vi "Get Functions Name.vi"(8 "error in (no error)":errorcluster, 11 "QDDialogList in":refnum<class "QDDialogList.lvclass">) -> (0 "error out":errorcluster, 2 "Functions Name":string[](array[string]), 3 "QDDialogList out":refnum<class "QDDialogList.lvclass">)   [LabVIEW 2015, in "QDDialogList.lvclass"]
uses:
  QDDialogList.lvclass
  QDDialogList.lvclass/QDDialogList.ctl
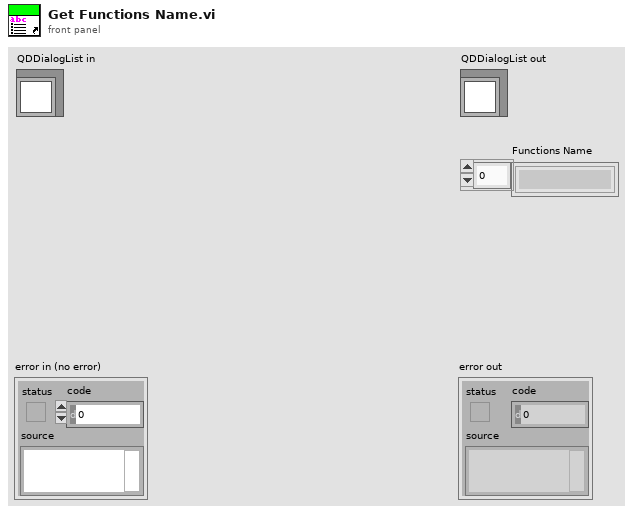
[diagram p1: front panel]
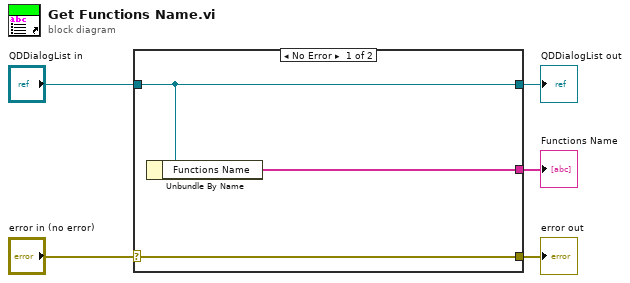
[diagram p0: block diagram]
diagram:
  n1 = case shown="No Error" "error in (no error)" {
    selector: "error in (no error)" -> [w8 w9]
    tunnel: [w8 w9] -> w4
    tunnel: [w7 w10] -> w2
    tunnel: "QDDialogList in" -> [w7 w10]
    tunnel: [w6 _] -> w1
    frame No Error {
      n2 = Unbundle By Name(w7) -> ("Functions Name"=w6:string[])
    }
    frame Error {
    }
  }
  "error out" <- w4
  "QDDialogList out" <- w2
  "Functions Name" <- w1
